vi "clientList.vi"(8 "error in (no error)":errorcluster, 9 "new client":refnum<k5>, 10 "Enum":enum16{"read", "write", "reset"}(ring), 11 "NetworkServer in":refnum<class "NetworkServer.lvclass">) -> (0 "error out":errorcluster, 1 "client":refnum<k5>, 2 "valid?":bool, 3 "NetworkServer out":refnum<class "NetworkServer.lvclass">)   [LabVIEW 2011, in "Hardware.lvlib" / "HWControllers.lvlib" / "NetworkServer.lvclass"]
uses:
  NetworkServer.lvclass
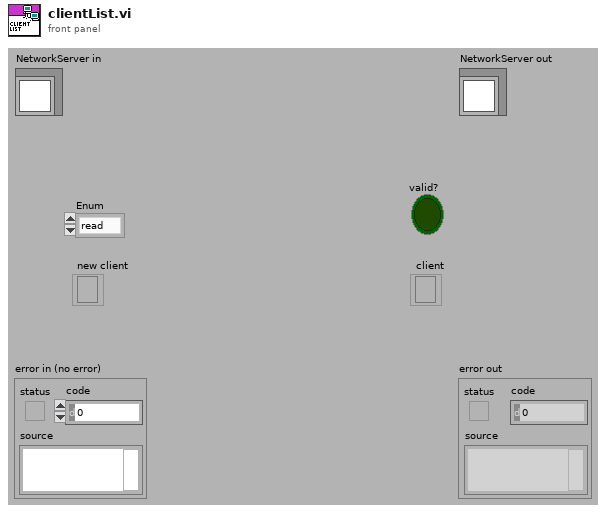
[diagram p1: front panel]
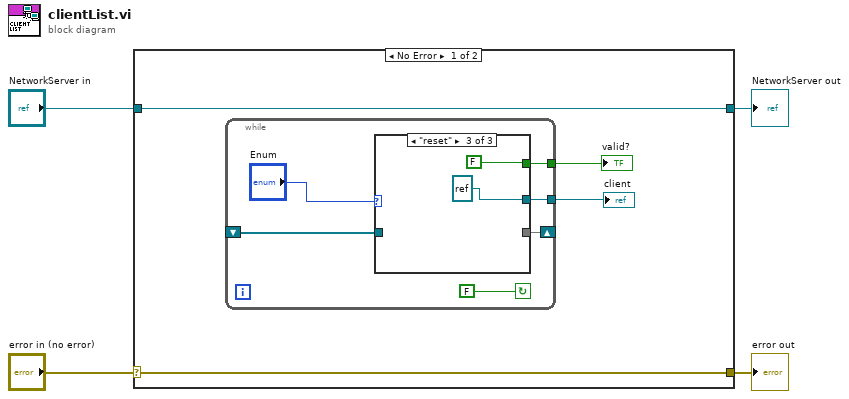
[diagram p0: block diagram]
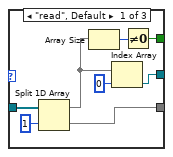
[diagram p2: hidden frame]
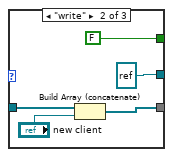
[diagram p3: hidden frame]
diagram:
  n1 = case shown="No Error" "error in (no error)" {
    selector: "error in (no error)" -> [w7 w31]
    tunnel: [w7 w31] -> w3
    tunnel: [w8 w30] -> w1
    tunnel: "NetworkServer in" -> [w8 w30]
    frame No Error {
      n2 = while {
        tunnel: [w11] -> w5
        tunnel: [w12] -> w6
        shift-left: _ -> [w13]
        shift-right: [w14] -> _
        stop <- FALSE continue-if-true
        n3 = case shown="\"reset\"" "Enum" {
          tunnel: [w20 w27 _] -> w14
          tunnel: w13 -> [w22 w26 _]
          tunnel: [w17 refnum<k5> refnum ("empty") refnum<k5> refnum ("empty")] -> w12
          tunnel: [w15 FALSE FALSE] -> w11
          frame "read", Default {
            n4 = Split 1D Array(array=w22, index=1) -> (first subarray=w18:refnum<k5>[], second subarray=w20:refnum<k5>[])
            n5 = Array Size(array=w18) -> (size(s)=w16:i32)
            n6 = Index Array(array=w18, index=0) -> (element=w17:refnum<k5>)
            n7 = Not Equal To 0?(x=w16) -> (x != 0?=w15:bool)
          }
          frame "write" {
            n8 = Build Array (concatenate)(w26, "new client") -> (w27:refnum<k5>[])
          }
          frame "reset" {
          }
        }
      }
      "client" <- w6
      "valid?" <- w5
    }
    frame Error {
    }
  }
  "error out" <- w3
  "NetworkServer out" <- w1
